vi "AttrSetMask.vi"(7 "error in":errorcluster, 9 "Value":u32, 10 "CanHandleIn":T1) -> (0 "error out":errorcluster, 3 "CanHandleOut":T1)   [LabVIEW 2011, in "Konvolucio MCAN120803.lvlib"]
uses:
  <instrlib>/Konvolucio MCAN120803/Konvolucio MCAN120803.lvlib
  <instrlib>/Konvolucio MCAN120803/Types/CanHandleType.ctl
  C:/Program Files/National Instruments/LabVIEW 2011/instr.lib/Konvolucio MCAN120803/Private/Konvolucio.MCAN120803.API.dll
  Private/Konvolucio.MCAN120803.API.dll
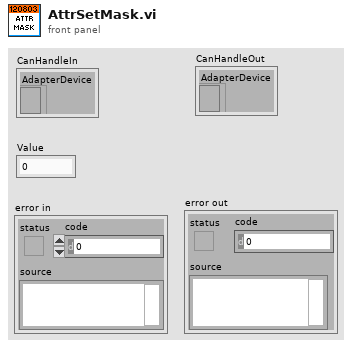
[diagram p1: front panel]
types:
  T1 = typedef "Konvolucio MCAN120803.lvlib/CanHandleType.ctl" = cluster{"AdapterDevice":refnum<k24>}
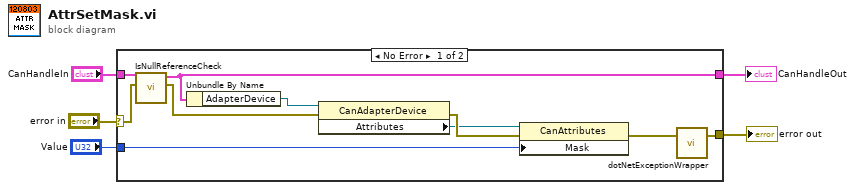
[diagram p0: block diagram]
diagram:
  n1 = case shown="No Error" "error in" {
    selector: "error in" -> [w10 w17]
    tunnel: [w14 w17] -> w5
    tunnel: "Value" -> [w15 _]
    tunnel: "CanHandleIn" -> [w11 w16]
    tunnel: [w12 w16] -> w1
    frame No Error {
      n2 = call <instrlib>:"IsNullReferenceCheck.vi"("error in"=w10, "MCanHandleIn"=w11) -> ("error out"=w8:errorcluster, "MCanHandleOut"=w12:T1)  [unwired: 5 in]
      n3 = Unbundle By Name(w12) -> ("AdapterDevice"=w9:refnum<k24>)
      n4 = property class="CanAdapterDevice"(reference=w9, error in=w8) -> (error out=w7:errorcluster, "Attributes"=w6:refnum<k24>)  [unwired: 1 out]
      n5 = property class="CanAttributes"(reference=w6, error in=w7, "Mask"=w15) -> (error out=w13:errorcluster)  [unwired: 1 out]
      n6 = call <instrlib>:"dotNetExceptionWrapper.vi"("error in"=w13) -> ("error out"=w14:errorcluster)  [unwired: 2 in]
    }
    frame Error {
    }
  }
  "error out" <- w5
  "CanHandleOut" <- w1
